vi "Subscribe.vi"(8 "error in (no error)":errorcluster, 10 "Topic Subscriptions":T1[](array[typedef]), 11 "MQTT_Base in":refnum<class "MQTT_Base.lvclass">) -> (0 "error out":errorcluster, 3 "MQTT_Base out":refnum<class "MQTT_Base.lvclass">)   [LabVIEW 2013, in "MQTT Server.lvlib" / "MQTT_Base.lvclass"]
uses:
  MQTT_Base.lvclass
  Control Packets/SUBSCRIBE/Topic Subscription -- cluster.ctl
  Control Packets/ControlPacket/QualityOfService -- enum.ctl
  Control Packets/SUBSCRIBE/SUBSCRIBE.lvclass
  Control Packets/ControlPacket/ControlPacket.lvclass
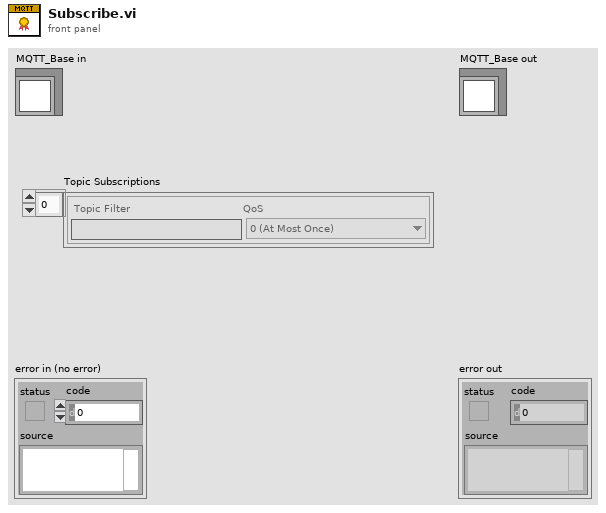
[diagram p1: front panel]
types:
  T1 = typedef "SUBSCRIBE.lvclass/Topic Subscription -- cluster.ctl" = cluster{"Topic Filter":string, "QoS":T2}
  T2 = typedef "ControlPacket.lvclass/QualityOfService -- enum.ctl" = enum16{"0 (At Most Once)", "1 (At Least Once)", "2 (Exactly Once)"}
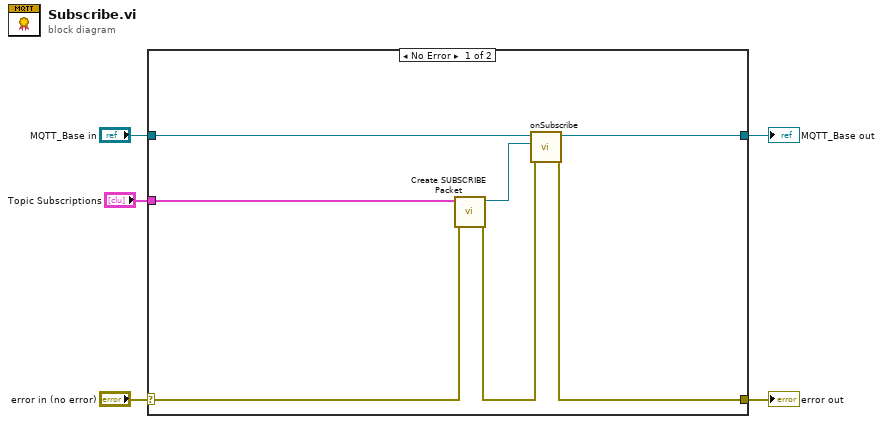
[diagram p0: block diagram]
diagram:
  n1 = case shown="No Error" "error in (no error)" {
    selector: "error in (no error)" -> [w7 w14]
    tunnel: [w10 w14] -> w4
    tunnel: [w11 w13] -> w2
    tunnel: "MQTT_Base in" -> [w12 w13]
    tunnel: "Topic Subscriptions" -> [w6 _]
    frame No Error {
      n2 = call "Create SUBSCRIBE Packet.vi"("error in (no error)"=w7, "Topic Subscriptions"=w6) -> ("error out"=w8:errorcluster, "SUBSCRIBE out"=w9:refnum<class "SUBSCRIBE.lvclass">)  [unwired: 8 in]
      n3 = call-dynamic "onSubscribe.vi"("error in (no error)"=w8, "SUBSCRIBE"=w9, "MQTT_Base in"=w12) -> ("error out"=w10:errorcluster, "MQTT_Base out"=w11:refnum<class "MQTT_Base.lvclass">)  [unwired: 7 in]
    }
    frame Error {
    }
  }
  "error out" <- w4
  "MQTT_Base out" <- w2
